vi "CTRE_Phoenix_CANdle_GetStatus.vi"(0 "CTRE_CANdle_DeviceRef":T1, 11 "error in":errorcluster) -> (4 "CTRE_CANdle_DeviceRef":T1, 6 "Bus Voltage":dbl, 8 "5V Rail Voltage":dbl, 10 "Current (amps)":dbl, 14 "Temperature (C)":dbl, 15 "error out":errorcluster)   [LabVIEW 2020]
doc: "Returns Output and Status of the CANdle.\n\n<b>Bus Voltage</b> is the input voltage to the CANdle.\n<b>5V Rail Voltage</b> is the current output voltage of the 5V rail.\n<b>Current (amps)</b> is the current draw through the output ground.\n<b>Temperature (C)</b> is the current temperature as measured by CANdle's processor."
uses:
  <vilib>/Rock Robotics/WPI/ThirdParty/Phoenix-LabVIEW/CANdle/Controls/CTRE_Phoenix_CANdle_DeviceRef.ctl
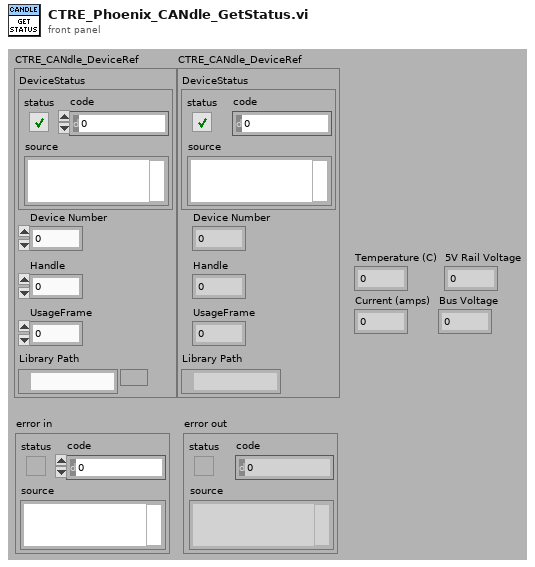
[diagram p1: front panel]
types:
  T1 = typedef "CTRE_Phoenix_CANdle_DeviceRef.ctl" = cluster{"DeviceStatus":errorcluster, "Device Number":u8, "Handle":u64, "UsageFrame":u32, "Library Path":path}
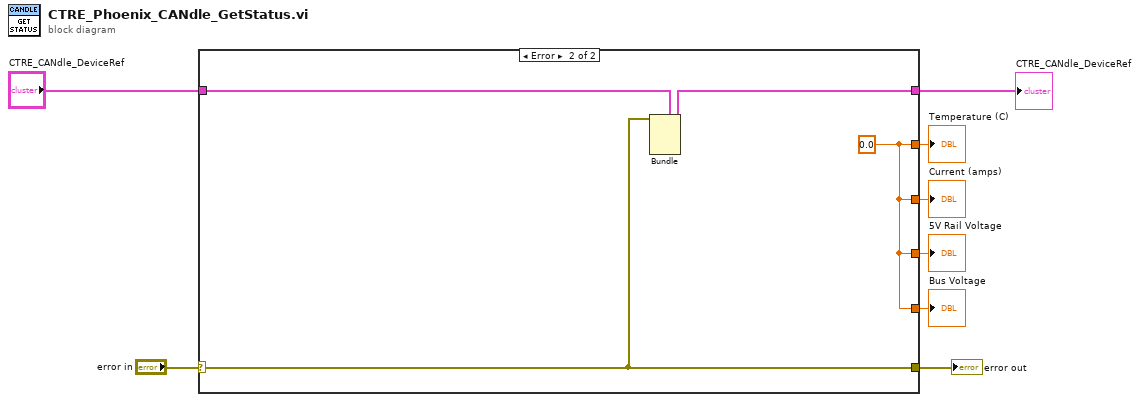
[diagram p0: block diagram]
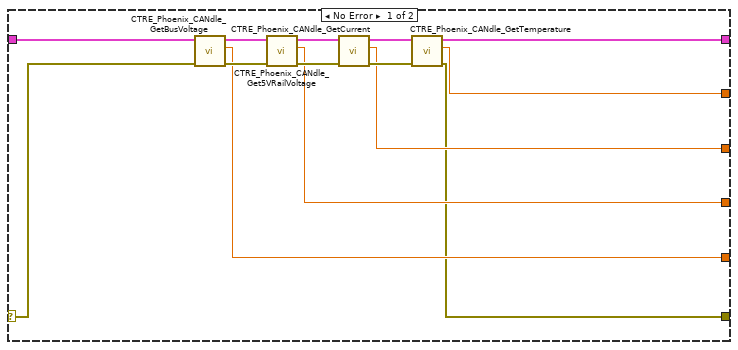
[diagram p2: hidden frame]
diagram:
  n1 = case shown="Error" "error in" {
    selector: "error in" -> [w21 w25]
    tunnel: "CTRE_CANdle_DeviceRef" -> [w22 w26]
    tunnel: [w9 w25] -> w8
    tunnel: [w14 w24] -> w5
    tunnel: [w13 w23] -> w1
    tunnel: [w12 w23] -> w2
    tunnel: [w11 w23] -> w3
    tunnel: [w10 w23] -> w4
    frame No Error {
      n2 = call <vilib>:"CTRE_Phoenix_CANdle_GetBusVoltage.vi"("error in"=w21, "CTRE_CANdle_DeviceRef"=w22) -> ("error out"=w20:errorcluster, "Bus Voltage"=w13:dbl, "CTRE_CANdle_DeviceRef"=w17:T1)  [unwired: 7 in]
      n3 = call <vilib>:"CTRE_Phoenix_CANdle_Get5VRailVoltage.vi"("error in"=w20, "CTRE_CANdle_DeviceRef"=w17) -> ("error out"=w19:errorcluster, "5V Rail Voltage"=w12:dbl, "CTRE_CANdle_DeviceRef"=w16:T1)  [unwired: 7 in]
      n4 = call <vilib>:"CTRE_Phoenix_CANdle_GetCurrent.vi"("error in"=w19, "CTRE_CANdle_DeviceRef"=w16) -> ("error out"=w18:errorcluster, "Current (amps)"=w11:dbl, "CTRE_CANdle_DeviceRef"=w15:T1)  [unwired: 7 in]
      n5 = call <vilib>:"CTRE_Phoenix_CANdle_GetTemperature.vi"("error in"=w18, "CTRE_CANdle_DeviceRef"=w15) -> ("error out"=w9:errorcluster, "Temperature (C)"=w10:dbl, "CTRE_CANdle_DeviceRef"=w14:T1)  [unwired: 7 in]
    }
    frame Error {
      w23 = 0.0 ("Position (Raw Sensor Units)")
      n6 = Bundle(cluster=w26, "DeviceStatus"=w25) -> (w24:T1)  [unwired: 4 in]
    }
  }
  "error out" <- w8
  "CTRE_CANdle_DeviceRef" <- w5
  "Temperature (C)" <- w4
  "Current (amps)" <- w3
  "5V Rail Voltage" <- w2
  "Bus Voltage" <- w1
